vi "waves.vi"() -> ()   [LabVIEW 2018]
panel:
  in  "resistor 2":dbl format="%#_6p"
  in  "capacitor 2":dbl format="%#_6p"
  out "time\nconstant 2":dbl format="%#_6p"
  in  "Vin 2":dbl format="%#_6p"
  out "VC(t) 2":dbl[](array[numeric])
  out "capacitance discharging":cluster{dbl, dbl, dbl[]}(graph)
  out "time\nconstant":dbl format="%#_6p"
  in  "Vin":dbl format="%#_6p"
  in  "capacitor":dbl format="%#_6p"
  in  "resistor":dbl format="%#_6p"
  out "VC(t)":dbl[](array[numeric])
  out "capacitance charging":cluster{dbl, dbl, dbl[]}(graph)
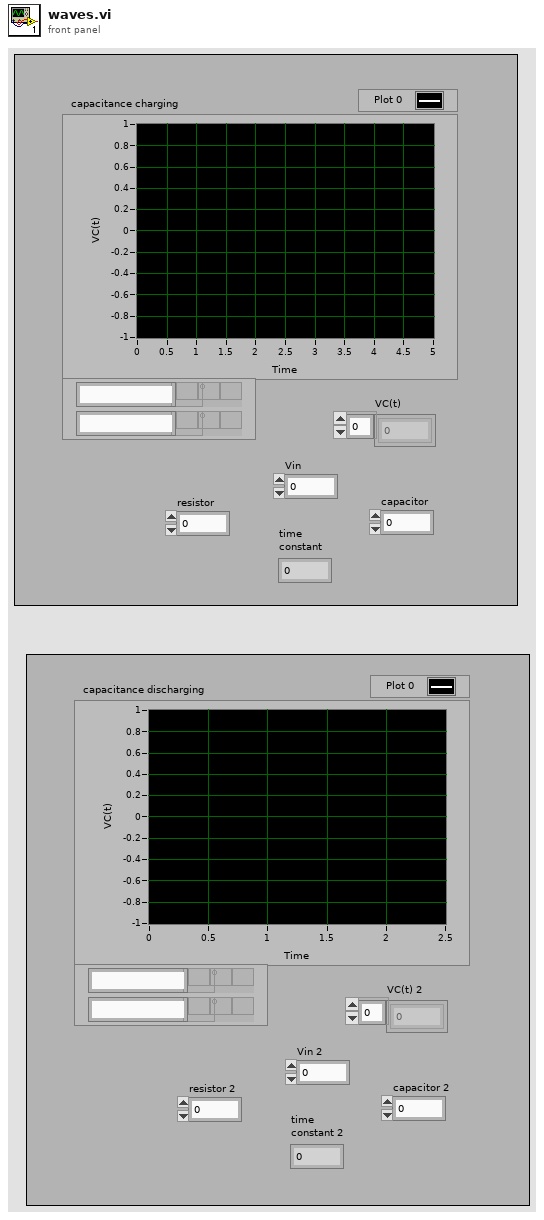
[diagram p1: front panel]
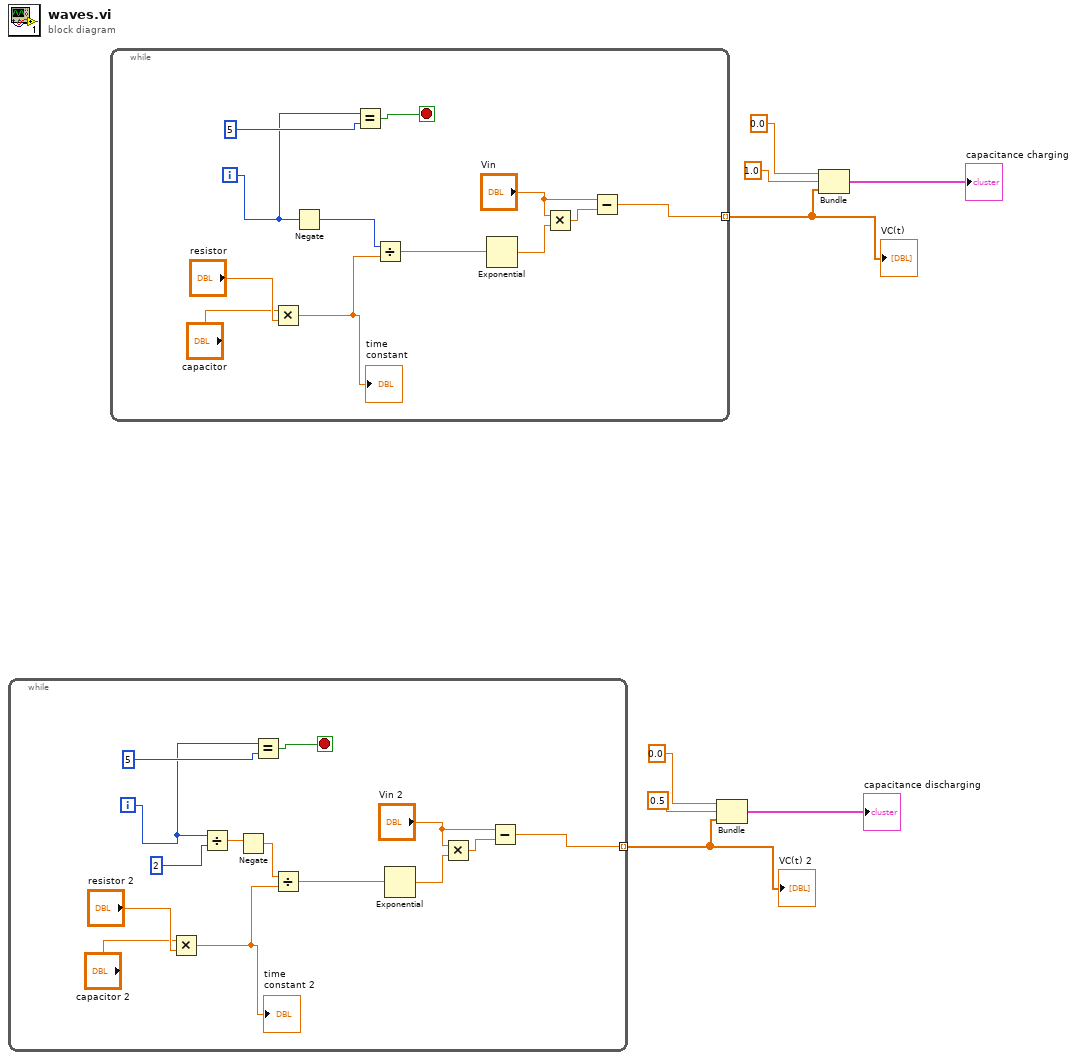
[diagram p0: block diagram]
diagram:
  n1 = while {
    tunnel: [w12] -> w1 mode=indexing
    i -> [w10]
    stop <- w19 stop-if-true
    n2 = Multiply(x="capacitor 2", y="resistor 2") -> (x*y=w20:dbl)
    "time\nconstant 2" <- w20
    n3 = Divide(x=w10, y=2) -> (x/y=w11:dbl)
    n4 = Negate(x=w11) -> (-x=w17:dbl)
    n5 = Equal?(x=w10, y=5) -> (x = y?=w19:bool)
    n6 = Divide(x=w17, y=w20) -> (x/y=w16:dbl)
    n7 = Exponential(1:w16) -> (0:w15:dbl)
    n8 = Multiply(x="Vin 2", y=w15) -> (x*y=w14:dbl)
    n9 = Subtract(x="Vin 2", y=w14) -> (x-y=w12:dbl)
  }
  "VC(t) 2" <- w1
  n10 = while {
    tunnel: [w23] -> w5 mode=indexing
    i -> [w29]
    stop <- w31 stop-if-true
    n11 = Multiply(x="capacitor", y="resistor") -> (x*y=w32:dbl)
    "time\nconstant" <- w32
    n12 = Negate(x=w29) -> (-x=w28:i32)
    n13 = Equal?(x=w29, y=5) -> (x = y?=w31:bool)
    n14 = Divide(x=w28, y=w32) -> (x/y=w27:dbl)
    n15 = Exponential(1:w27) -> (0:w26:dbl)
    n16 = Multiply(x="Vin", y=w26) -> (x*y=w25:dbl)
    n17 = Subtract(x="Vin", y=w25) -> (x-y=w23:dbl)
  }
  "VC(t)" <- w5
  n18 = Bundle(0.0, 0.5, w1) -> (→"capacitance discharging":cluster{dbl, dbl, dbl[]})  [unwired: 1 in]
  n19 = Bundle(0.0, 1.0, w5) -> (→"capacitance charging":cluster{dbl, dbl, dbl[]})  [unwired: 1 in]
